vi "Launch.vi"(8 "error in (no error)":errorcluster, 10 "Show Front Panel? (F)":bool, 11 "API in":refnum<class "Interface.lvclass">) -> (0 "error out":errorcluster, 1 "Already Launched":bool, 3 "API out":refnum<class "Interface.lvclass">)   [LabVIEW 2018, in "Scripting.lvlib" / "Actor.lvlib" / "Interface.lvclass"]
uses:
  Interface.lvclass
  Interface.lvclass/Interface.ctl
  Front-Panel State.ctl
  Actor.lvclass
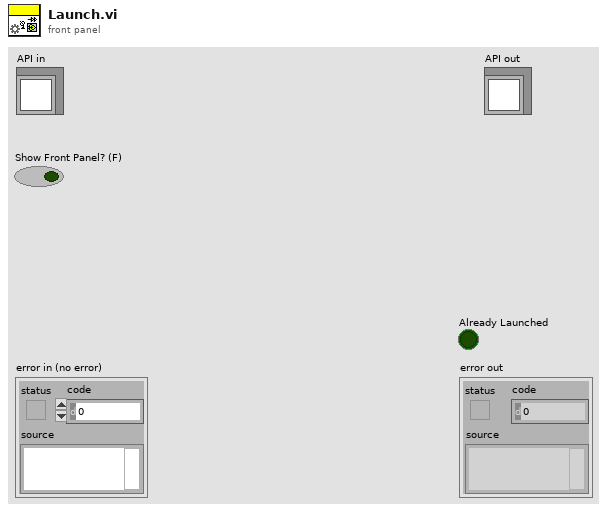
[diagram p1: front panel]
types:
  T1 = typedef "Scripting.lvlib/Actor.lvlib/Actor.lvclass/Front-Panel State.ctl" = enum16{"Don't Show", "Show"}
  T2 = typedef "Scripting.lvlib/Actor.lvlib/Interface.lvclass/API-Data.ctl" = cluster{"Launch":refnum<notifier>, "Actor Stopped":cluster{"Enqueuer":refnum<user-event>, "Message":refnum<event-registration>}, "Requests":T3}
  T3 = typedef "Scripting.lvlib/Actor.lvlib/Actor.lvclass/Request-Enqueuers.ctl" = cluster{"Get State":refnum<user-event>, "Stop":refnum<user-event>}
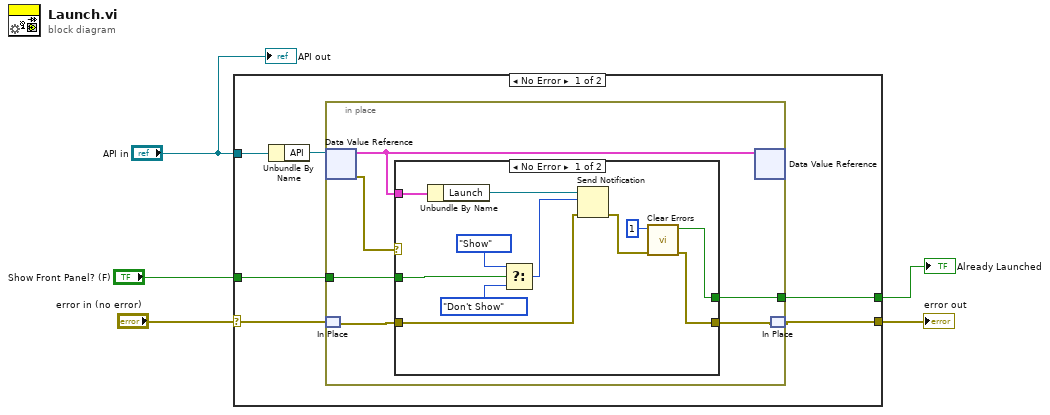
[diagram p0: block diagram]
diagram:
  n1 = case shown="No Error" "error in (no error)" {
    selector: "error in (no error)" -> [w8 w30]
    tunnel: [w7 w30] -> w4
    tunnel: [w11 _] -> w3
    tunnel: "Show Front Panel? (F)" -> [w10 _]
    tunnel: "API in" -> [w9 _]
    frame No Error {
      n2 = Unbundle By Name(w9) -> ("API"=w6:refnum<data-value>)
      n3 = in-place {
        in-place-border: [w17] -> w11
        in-place-border: w10 -> [w16]
        n4 = in-place-dvr #1(w6) -> (w13:T2, w12:errorcluster)
        n5 = in-place-match #2(w8) -> (w15:errorcluster)
        n6 = case shown="No Error" w12 {
          selector: w12 -> [_ w29]
          tunnel: [w28 _] -> w17
          tunnel: w16 -> [w27 _]
          tunnel: w15 -> [w20 _]
          tunnel: [w19 w29] -> w14
          tunnel: w13 -> [w18 _]
          frame No Error {
            n7 = Unbundle By Name(w18) -> ("Launch"=w25:refnum<notifier>)
            n8 = Select(t=Front-Panel_State."Show" ("notification"), s=w27, f=Front-Panel_State."Don't Show" ("notification")) -> (s? t:f=w21:T1)
            n9 = Send Notification(notification=w21, notifier=w25, error in (no error)=w20) -> (error out=w24:errorcluster)  [unwired: 1 out]
            n10 = call <vilib>:"Clear Errors.vi"("error in (no error)"=w24, "specific error code to clear (0: all)"=1) -> ("error out"=w19:errorcluster, "specific error cleared?"=w28:bool)  [unwired: 4 in]
          }
          frame Error {
          }
        }
        n11 = in-place-dvr #1(w13) -> ()  [unwired: 2 out]
        n12 = in-place-match #2(w14) -> (w7:errorcluster)
      }
    }
    frame Error {
    }
  }
  "error out" <- w4
  "Already Launched" <- w3
  "API out" <- "API in"
